vi "Restore Panel Config.vi"(8 "error in (no error)":errorcluster, 10 "EditPanel API in":refnum<class "EditPanel API.lvclass">, 11 "Console Reply in":refnum<class "Console Reply.lvclass">) -> (0 "error out":errorcluster, 2 "EditPanel API out":refnum<class "EditPanel API.lvclass">, 3 "Console Reply out":refnum<class "Console Reply.lvclass">)   [LabVIEW 2015, in "EditPanel API.lvlib" / "Console Reply.lvclass"]
uses:
  Console Reply.lvclass
  EditPanel_class/EditPanel API.lvclass
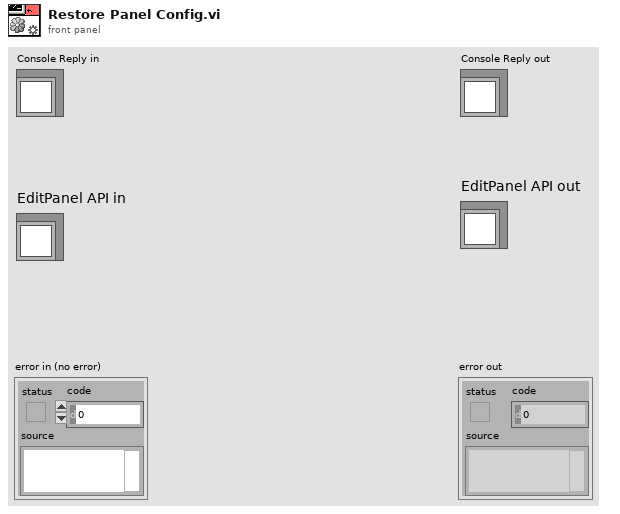
[diagram p1: front panel]
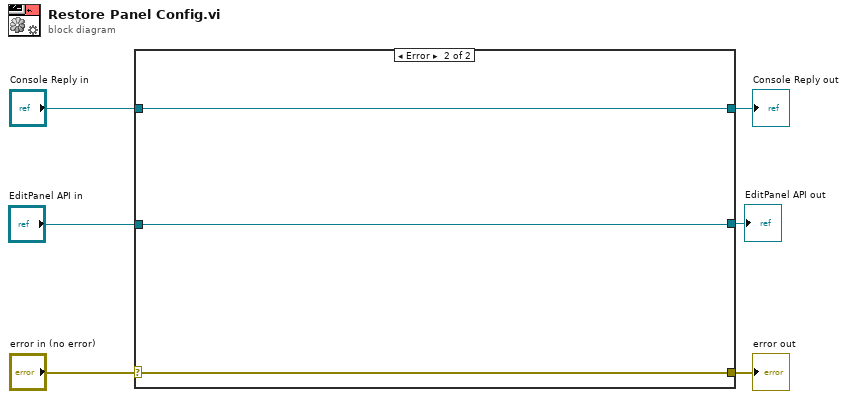
[diagram p0: block diagram]
diagram:
  n1 = case shown="Error" "error in (no error)" {
    selector: "error in (no error)" -> [w8 w12]
    tunnel: [w8 w12] -> w5
    tunnel: [w9 w11] -> w3
    tunnel: "Console Reply in" -> [w9 w11]
    tunnel: [w7 w10] -> w1
    tunnel: "EditPanel API in" -> [w7 w10]
    frame No Error {
    }
    frame Error {
    }
  }
  "error out" <- w5
  "Console Reply out" <- w3
  "EditPanel API out" <- w1
